vi "hasPacketIdentifier.vi"(11 "CONNECT in":refnum<class "CONNECT.lvclass">) -> (2 "As Packet Identifier":bool, 3 "CONNECT out":refnum<class "CONNECT.lvclass">)   [LabVIEW 2013, in "CONNECT.lvclass"]
uses:
  CONNECT.lvclass
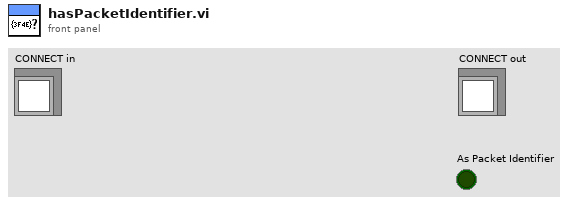
[diagram p1: front panel]
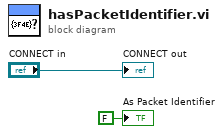
[diagram p0: block diagram]
diagram:
  "CONNECT out" <- "CONNECT in"
  "As Packet Identifier" <- FALSE ("As Packet Identifier")
